vi "Handle Command.vi"(8 "error in":errorcluster, 10 "Exe Write in":refnum<class "Exe Write.lvclass">, 11 "Object In":refnum<class>) -> (0 "error out":errorcluster, 1 "Command Succesful?":bool, 2 "Exe Write out":refnum<class "Exe Write.lvclass">, 3 "Object Out":refnum<class>)   [LabVIEW 2014, in "File Library.lvlib" / "Exe Write.lvclass"]
doc: "Execute the file write. This method uses a strategy pattern that is determined by the Exe Write object and the Saving File Message Object."
uses:
  Exe Write.lvclass
  File Actor.lvclass
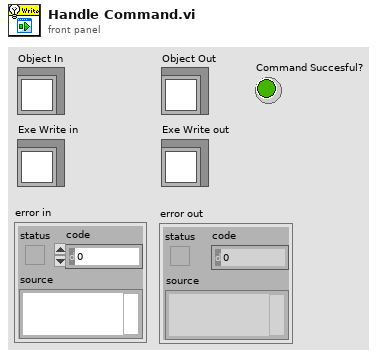
[diagram p1: front panel]
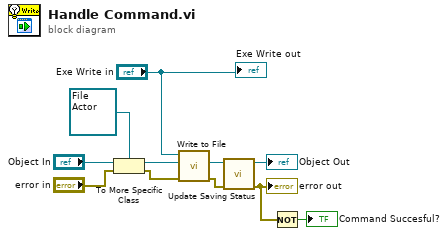
[diagram p0: block diagram]
diagram:
  n1 = To More Specific Class(target class=refnum<class "File Actor.lvclass"> refnum ("File Library.lvlib:File Actor"), reference="Object In", error in="error in") -> (specific class reference=w7:refnum<class "File Actor.lvclass">, error out=w5:errorcluster)
  n2 = call-dynamic "Write to File.vi"("error in"=w5, "File Actor In"=w7, "Exe Write in"="Exe Write in") -> ("error out"=w4:errorcluster, "File Actor Out"=w6:refnum<class "File Actor.lvclass">)  [unwired: 7 in]
  n3 = call "Update Saving Status.vi"("error in"=w4, "File Actor in"=w6) -> ("error out"=w2:errorcluster, "File Actor out"=→"Object Out":refnum<class "File Actor.lvclass">)  [unwired: 8 in]
  "error out" <- w2
  n4 = Not(x=w2) -> (.not. x?=→"Command Succesful?":bool)
  "Exe Write out" <- "Exe Write in"
